vi "Digitizer Analyze_SNR.vi"(6 "frequency range":T1={"start frequency"=-1.0, "stop frequency"=-1.0}, 7 "Pins":string[](array[string])=["Xout"], 8 "error in":errorcluster, 9 "Published Data Id":string[](array[string]), 10 "Waveform Data In":waveform(dbl)[](array[waveform])=[{"t0"=timestamp(3637030365.2340937 s since 1904-01-01), "dt"=3.3333333333333334e-08, "Y"=array[5343 elements]}, {"t0"=timestamp(3637030365.2340937 s since 1904-01-01), "dt"=3.3333333333333334e-08, "Y"=array[5343 elements]}], 11 "Semiconductor Module Context":T2) -> (0 "error out":errorcluster, 1 "Frequency (Hz)":dbl format="%.2f", 2 "SNR (dB)":dbl format="%.2f", 3 "Power (dBm)":dbl)   [LabVIEW 2014]
doc: "Example: Measurement Library\n\nRecommended Input Signal: 100 kHz, 2 Vpp, sine wave\n\nDevices Supported: Refer to NI Example Finders\n\nLabVIEW Description:\n\nThis example illustrates fetching scalar measurements from NI-SCOPE, such as period and rise time calculations. \n\nSome common horizontal and vertical parameters are configured for the oscilloscope. The property node is used to set the reference level units, and the low, middle and high reference levels. For more information about measurement library parameters, see the NI-SCOPE VI Reference Help file. \n\nAfter the Read VI is called to acquire a waveform, the Fetch Measurement Stats VI is used to perform the desired scalar measurement analysis on the waveform. NI-SCOPE keeps a history of each measurement's results, which allows it to retrieve the statistics computed over multiple acquisitions. These statistics include the mean, standard deviation, min, max and number of acquisitions used in the statistics. The statistics are updated once per acquisition when the measurement is fetched. The Clear Stats VI clears this history."
uses:
  <vilib>/NI_TestStand_SemiconductorModule/NI_TestStand_Semiconductor_Module.lvlibp/PinMap/General/SemiconductorModuleContext.ctl
  <vilib>/NI_TestStand_SemiconductorModule/NI_TestStand_Semiconductor_Module.lvlibp/PinMap/General/NIInstrumentTypeIDs.ctl
  <vilib>/addons/_NISVFA/_Shared subVIs/Controls/svc_Window.ctl
  <vilib>/addons/_NISVFA/_Baseband FFT/SVFA FFT Spectrum (Complex) (1 Ch).vi
  <vilib>/addons/_NISVFA/_Spectrum Processing/SVFA Unit Conversion (Complex) (1 Ch).vi
  <vilib>/NI_TestStand_SemiconductorModule/NI_TestStand_Semiconductor_Module.lvlibp/PinMap/General/Publish/PublishDataDoubleFunctionalTest.vi
  <vilib>/NI_TestStand_SemiconductorModule/NI_TestStand_Semiconductor_Module.lvlibp
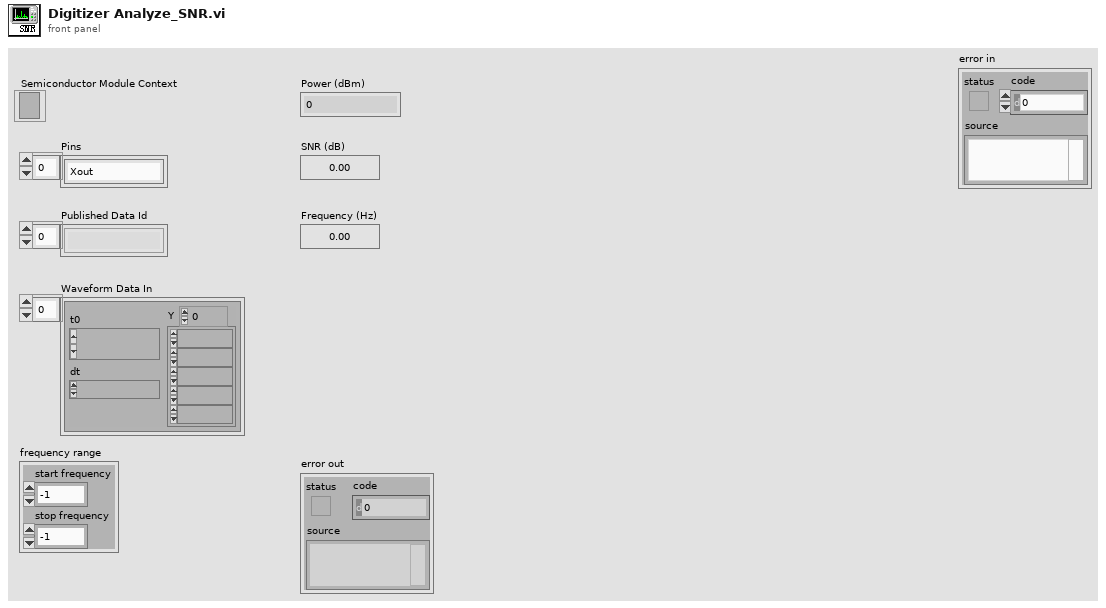
[diagram p1: front panel]
types:
  T1 = cluster{"start frequency":dbl, "stop frequency":dbl}
  T2 = typedef "NI_TestStand_Semiconductor_Module.lvlibp/SemiconductorModuleContext.ctl" = refnum<k7>
  T3 = typedef "svc_Window.ctl" = u32
  T4 = typedef "NI_TestStand_Semiconductor_Module.lvlibp/NIInstrumentTypeIDs.ctl" = string
  T5 = cluster{"linear/dB":enum16{"no change", "linear", "dB"}, "dB reference (0: no change)":dbl, "power/magnitude":enum16{"no change", "power", "magnitude"}, "view":enum16{"no change", "rms", "peak", "peak-peak"}}
  T6 = typedef "svc_Spectrum Info.ctl" = cluster{"channel name":string, "description":string, "x-axis units":T7, "spectral info":cluster{"spectrum type":T8, "linear/dB":enum16{"linear", "dB"}, "window":u16, "window size":i32, "FFT size":i32}, "engineering units":T9, "custom label":string, "dB reference [EU]":dbl, "peak units":enum16{"rms", "peak", "peak-peak"}, "weighting filter":T10, "spectral density?":bool, "unit label":string, "spectrum skewed?":bool, "complimentary spectrum units":T11}
  T7 = typedef "svc_X-Axis Units.ctl" = u16
  T8 = typedef "svc_Spectrum Type.ctl" = enum16{"FFT Spectrum [complex]", "Amplitude [Magnitude]", "Power [Magnitude^2]", "Cross Spectrum [complex]", "Frequency Response [Complex]"}
  T9 = typedef "svc_Engineering Units Text Ring.ctl" = u16
  T10 = typedef "svc_Weighting Filter Text Ring.ctl" = u16
  T11 = typedef "svc_Complimentary Spectrum Units.ctl" = enum16{"none", "radians", "degrees", "cycles", "imaginary"}
  T12 = cluster{"complex spectrum response":cluster{"f0":dbl, "df":dbl, "complex spectrum":cdb[]}, "spectrum info":T6}
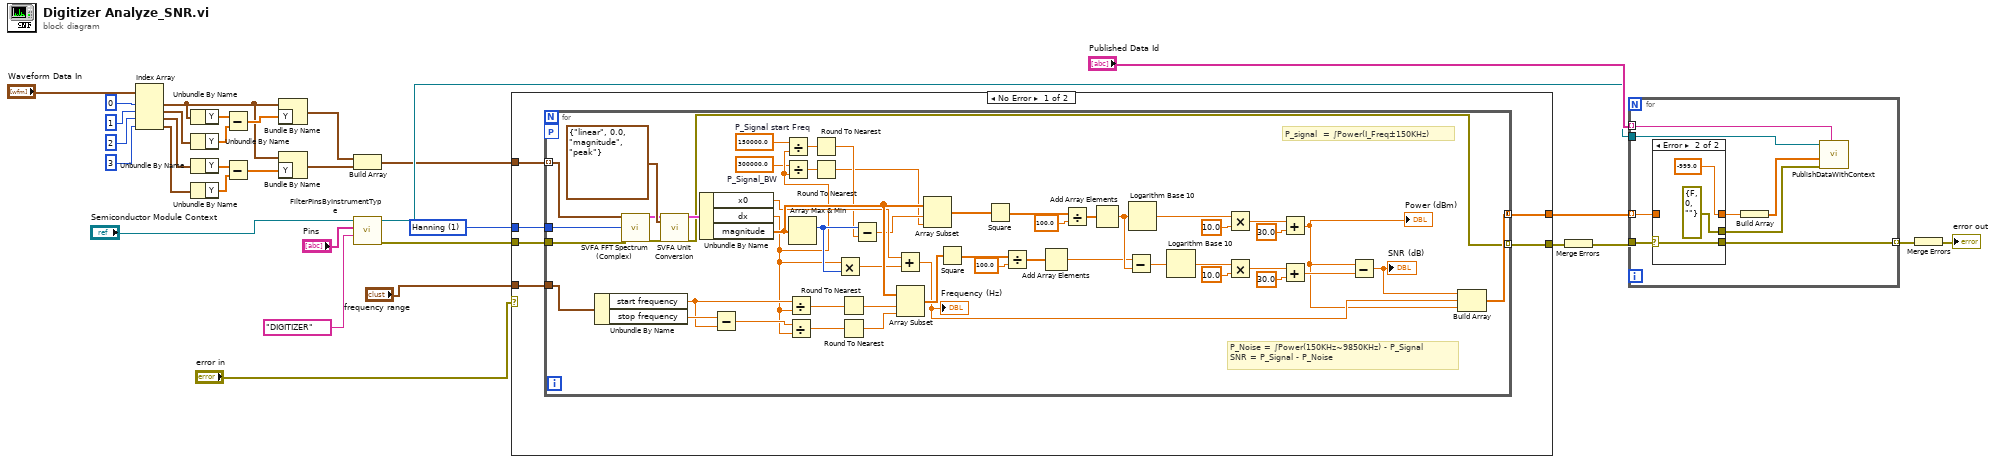
[diagram p0: block diagram]
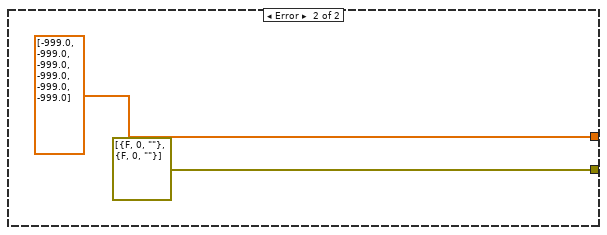
[diagram p2: hidden frame]
diagram:
  w28 = T3 1 items=["None"=0, "Hanning"=1, "Hamming"=2, "Blackman-Harris"=3, "Exact Blackman"=4, "Blackman"=5, "Flat Top"=6, "4 Term B-Harris "=7, "7 Term B-Harris"=8, "Low Sidelobe"=9, "Force"=64, "Exponential"=65, "Blackman Nuttall"=11, "Triangle"=30, "Bartlett-Hanning"=31, "Bohman"=32, "Parzen"=33, "Welch"=34, "Kaiser"=60, "Dolph-Chebyshev"=61, "Gaussian"=62] ("window")
  n1 = Index Array(array="Waveform Data In", index #1=0 ("index"), index #2=1 ("index"), index #3=2 ("index"), index #4=3 ("index")) -> (element #1=w10:waveform(dbl), element #2=w18:waveform(dbl), element #3=w17:waveform(dbl), element #4=w16:waveform(dbl))
  n2 = Unbundle By Name(w10) -> ("Y"=w24:dbl[])
  n3 = Unbundle By Name(w18) -> ("Y"=w23:dbl[])
  n4 = Unbundle By Name(w17) -> ("Y"=w13:dbl[])
  n5 = Unbundle By Name(w16) -> ("Y"=w12:dbl[])
  n6 = Subtract(x=w24, y=w23) -> (x-y=w29:dbl[])
  n7 = Subtract(x=w13, y=w12) -> (x-y=w11:dbl[])
  n8 = Bundle By Name(cluster=w10, "Y"=w29) -> (w9:waveform(dbl))
  n9 = Bundle By Name(cluster=w10, "Y"=w11) -> (w8:waveform(dbl))
  n10 = Build Array(w9, w8) -> (w7:waveform(dbl)[])
  n11 = call <vilib>:"FilterPinsByInstrumentType.vi"("Instrument Type Id"=T4 "DIGITIZER", "Pins"="Pins", "Semiconductor Module Context"="Semiconductor Module Context") -> ("error out"=w19:errorcluster, "Semiconductor Module Context Out"=w20:T2)  [unwired: 6 in, 1 out]
  n12 = case shown="No Error" "error in" {
    tunnel: w28 -> [w38 _]
    tunnel: [w33 dbl[] [-999.0, -999.0, -999.0, -999.0, -999.0, -999.0]] -> w21
    tunnel: w19 -> [w37 _]
    tunnel: "frequency range" -> [w36 _]
    tunnel: w7 -> [w35 _]
    tunnel: [w34 errorcluster[] [{"status"=FALSE, "code"=0, "source"=""}, {"status"=FALSE, "code"=0, "source"=""}]] -> w4
    frame No Error {
      n13 = for {
        tunnel: w35 -> [w57] mode=indexing
        tunnel: w38 -> [w58]
        tunnel: [w90] -> w33 mode=concatenating
        tunnel: w36 -> [w53]
        workers-P: _ -> [_]
        tunnel: w37 -> [w59]
        tunnel: [w60] -> w34 mode=indexing
        w41 = 300000.0  # P_Signal_BW
        w42 = 150000.0  # P_Signal start Freq
        # "P_Noise = ∫Power(150KHz~9850KHz) - P_Signal\nSNR = P_Signal - P_Noise"
        # "P_signal  = ∫Power(I_Freq±150KHz)"
        n14 = Unbundle By Name(w53) -> ("start frequency"=w49:dbl, "stop frequency"=w50:dbl)
        n15 = call-poly <vilib>:"SVFA FFT Spectrum (Complex).vi"("scaled signal [EU]"=w57, "window"=w58, "error in"=w59) -> ("complex spectrum"=w61:T12, "error out"=w62:errorcluster)  [unwired: 13 in, 2 out]
        n16 = call-poly <vilib>:"SVFA Unit Conversion.vi"("complex spectrum"=w61, "desired scaling"=T5 {"linear/dB"=enum."linear", "dB reference (0: no change)"=0.0, "power/magnitude"=enum."magnitude", "view"=enum."peak"}, "error in (no error)"=w62) -> ("converted spectrum"=w64:cluster{"x0":dbl, "dx":dbl, "magnitude":dbl[]}, "error out"=w60:errorcluster)  [unwired: 11 in, 4 out]
        n17 = Unbundle By Name(w64) -> ("x0"=w74:dbl, "dx"=w43:dbl, "magnitude"=w77:dbl[])
        n18 = Subtract(x=w50, y=w49) -> (x-y=w48:dbl)
        n19 = Divide(x=w42, y=w43) -> (x/y=w45:dbl)
        n20 = Divide(x=w41, y=w43) -> (x/y=w44:dbl)
        n21 = Divide(x=w49, y=w43) -> (x/y=w52:dbl)
        n22 = Divide(x=w48, y=w43) -> (x/y=w47:dbl)
        n23 = Array Max & Min(array=w77) -> (max index (indices)=w76:i32)  [unwired: 3 out]
        n24 = Round To Nearest(number=w45) -> (nearest integer value=w40:dbl)
        n25 = Round To Nearest(number=w44) -> (nearest integer value=w39:dbl)
        n26 = Multiply(x=w43, y=w76) -> (x*y=w75:dbl)
        n27 = Round To Nearest(number=w52) -> (nearest integer value=w51:dbl)
        n28 = Round To Nearest(number=w47) -> (nearest integer value=w46:dbl)
        n29 = Subtract(x=w76, y=w40) -> (x-y=w65:dbl)
        n30 = Add(x=w74, y=w75) -> (x+y=w55:dbl)
        "Frequency (Hz)" <- w55
        n31 = Array Subset(array=w77, index=w51, length=w46) -> (w85:dbl[])
        n32 = Array Subset(array=w77, index=w65, length=w39) -> (w66:dbl[])
        n33 = Square(x=w85) -> (x^2=w78:dbl[])
        n34 = Square(x=w66) -> (x^2=w67:dbl[])
        n35 = Divide(x=w78, y=100.0) -> (x/y=w80:dbl[])
        n36 = Add Array Elements(numeric array=w80) -> (sum=w86:dbl)
        n37 = Divide(x=w67, y=100.0) -> (x/y=w69:dbl[])
        n38 = Add Array Elements(numeric array=w69) -> (sum=w87:dbl)
        n39 = Subtract(x=w86, y=w87) -> (x-y=w88:dbl)
        n40 = Logarithm Base 10(1:w87) -> (0:w70:dbl)
        n41 = Logarithm Base 10(1:w88) -> (0:w81:dbl)
        n42 = Multiply(x=w70, y=10.0) -> (x*y=w72:dbl)
        n43 = Multiply(x=w81, y=10.0) -> (x*y=w83:dbl)
        n44 = Add(x=w72, y=30.0) -> (x+y=w54:dbl)
        "Power (dBm)" <- w54
        n45 = Add(x=w83, y=30.0) -> (x+y=w89:dbl)
        n46 = Subtract(x=w54, y=w89) -> (x-y=w56:dbl)
        "SNR (dB)" <- w56
        n47 = Build Array(w56, w55, w54) -> (w90:dbl[])
      }
    }
    frame Error {
    }
  }
  n48 = Merge Errors(w4) -> (w3:errorcluster)
  n49 = for {
    tunnel: "Published Data Id" -> [w100] mode=indexing
    tunnel: w21 -> [w97] mode=indexing
    tunnel: w20 -> [w99]
    tunnel: w3 -> [w98]
    tunnel: [w93] -> w6 mode=indexing
    n50 = case shown="Error" w98 {
      selector: w98 -> [w101 w103]
      tunnel: w97 -> [w102 _]
      tunnel: [w102 -999.0 ("detected fundamental\nfrequency [Hz]")] -> w96
      tunnel: [w101 errorcluster {"status"=FALSE, "code"=0, "source"=""} ("error IO")] -> w94
      tunnel: [w101 w103] -> w93
      frame No Error {
      }
      frame Error {
      }
    }
    n51 = Build Array(w96) -> (w95:dbl[])
    n52 = call-poly <vilib>:"PublishDataWithContext.vi"("Published Data Id"=w100, "error in (no error)"=w94, "Data In"=w95, "Semiconductor Module Context"=w99) -> ()  [unwired: 6 in, 2 out]
  }
  n53 = Merge Errors(w6) -> (→"error out":errorcluster)
